vi "tipshaping.vi"(8 "error in (no error)":errorcluster, 11 "Input":string="-286.640625n,21.171875n,-1.8n,20m,200m") -> (0 "error out":errorcluster, 3 "Output":string="-7.271E-9")   [LabVIEW 2019]
panel:
  out "size(s)":i32=5
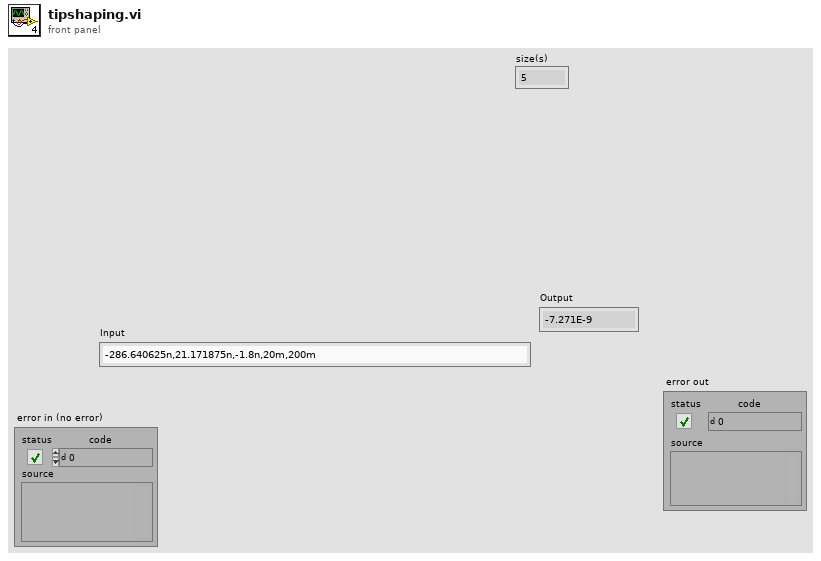
[diagram p1: front panel]
types:
  T1 = cluster{"TipLift":dbl, "Bias Settling Time":dbl, "Lift Height":dbl, "Lift Time 2":dbl, "Lifting Bias":dbl, "Lift Time 1":dbl}
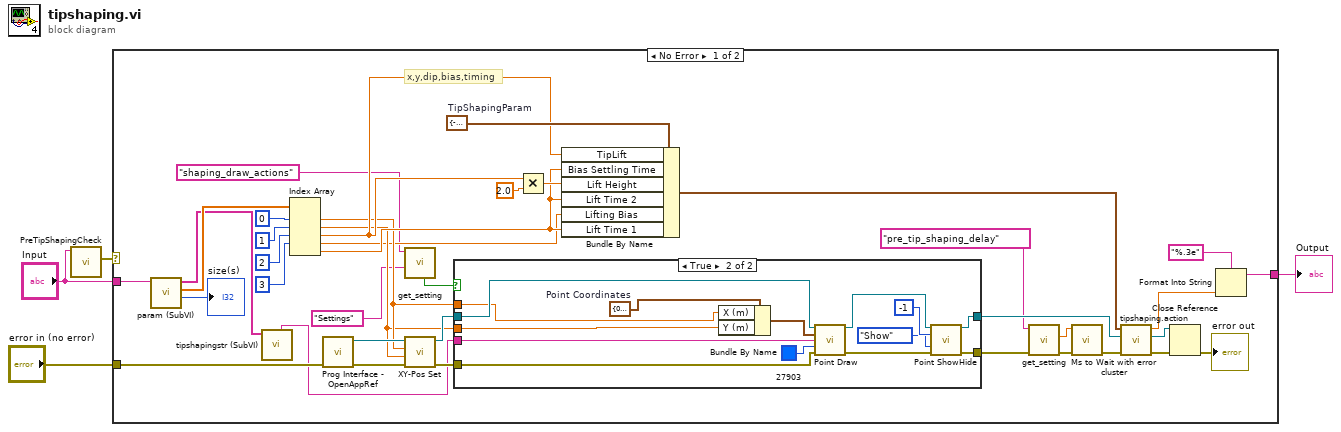
[diagram p0: block diagram]
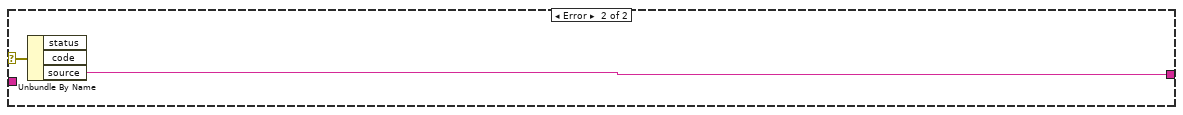
[diagram p3: hidden frame]
diagram:
  n1 = call "PreTipShapingCheck.vi"("Input"="Input") -> ("Error"=w1:errorcluster)  [unwired: 8 in, 2 out]
  n2 = case shown="No Error" w1 {
    selector: w1 -> [_ w60]
    tunnel: [w40 w59] -> w4
    tunnel: "error in (no error)" -> [w33 _]
    tunnel: "Input" -> [w18 _]
    frame No Error {
      w37 = T1 {"TipLift"=-2e-10, "Bias Settling Time"=0.09999999999999999, "Lift Height"=5e-09, "Lift Time 2"=0.2, "Lifting Bias"=2.0, "Lift Time 1"=0.2}  # TipShapingParam
      # "x,y,dip,bias,timing"
      n3 = call "param (SubVI).vi"("Input"=w18) -> ("num"=→"size(s)":i32, "parm"=w41:dbl[], "Array"=w19:string[])  [unwired: 8 in]
      n4 = call "tipshapingstr (SubVI).vi"("Array"=w19) -> ("String"=w20:string)  [unwired: 10 in]
      n5 = Index Array(array=w41, index #1=0 ("index"), index #2=1 ("index"), index #3=2 ("index"), index #4=3 ("index")) -> (element #1=w26:dbl, element #2=w25:dbl, element #3=w32:dbl, element #4=w13:dbl, element #5=w29:dbl)  [unwired: 1 in]
      n6 = call <userlib>:"Prog Interface - OpenAppRef.vi"("Error in (no error)"=w33) -> ("Error out"=w34:errorcluster, "Application reference"=w35:refnum<vi>)  [unwired: 5 in]
      n7 = call "get_setting.vi"("section"="Settings", "key"="shaping_draw_actions") -> ("Boolean"=w5:bool)  [unwired: 5 in, 4 out]
      n8 = call <userlib>:"XY-Pos Set.vi"("error in (no error)"=w34, "Y (m)"=w25, "X (m)"=w26, "Application ref in"=w35) -> ("error out"=w27:errorcluster, "Application ref out"=w28:refnum<vi>)  [unwired: 4 in]
      n9 = case shown="True" w5 {
        tunnel: w28 -> [w44 w58]
        tunnel: [w44 w55] -> w17
        tunnel: w27 -> [w43 w57]
        tunnel: [w43 w54] -> w11
        tunnel: w26 -> [_ w47]
        tunnel: w25 -> [_ w46]
        tunnel: w20 -> [_ w45]
        frame False {
        }
        frame True {
          w49 = cluster{"X (m)":sgl, "Y (m)":sgl} {"X (m)"=0.0, "Y (m)"=0.0}  # Point Coordinates
          n10 = Bundle By Name(cluster=w49, "X (m)"=w47, "Y (m)"=w46) -> (w48:cluster{"X (m)":sgl, "Y (m)":sgl})
          n11 = call <userlib>:"Point Draw.vi"("Application ref in"=w58, "Point Coordinates"=w48, "Text"=w45, "Color"=u32 27903, "error in (no error)"=w57) -> ("Application ref out"=w56:refnum<vi>, "error out"=w53:errorcluster)  [unwired: 9 in]
          n12 = call <userlib>:"Point ShowHide.vi"("Application ref in"=w56, "Point index (-1=All points)"=-1, "Show/Hide"=enum16{"Show", "Hide"}."Show", "error in (no error)"=w53) -> ("Application ref out"=w55:refnum<vi>, "error out"=w54:errorcluster)  [unwired: 10 in]
        }
      }
      n13 = Multiply(x=w32, y=2.0) -> (x*y=w31:dbl)
      n14 = Bundle By Name(cluster=w37, "TipLift"=w32, "Bias Settling Time"=w29, "Lift Height"=w31, "Lift Time 2"=w29, "Lifting Bias"=w13, "Lift Time 1"=w29) -> (w36:T1)
      n15 = call "get_setting.vi"("error in (no error)"=w11, "key"="pre_tip_shaping_delay") -> ("error out"=w10:errorcluster, "output 1"=w9:dbl)  [unwired: 5 in, 3 out]
      n16 = call <userlib>:"Ms to Wait with error cluster.vi"("error in (no error)"=w10, "milliseconds to wait"=w9) -> ("error out"=w12:errorcluster)  [unwired: 4 in, 1 out]
      n17 = call "tipshaping.action.vi"("Error in (no error)"=w12, "Application reference"=w17, "TipShapingParam"=w36) -> ("error out"=w15:errorcluster, "Application ref out"=w16:refnum<vi>, "dz"=w39:sgl)  [unwired: 6 in]
      n18 = Close Reference(reference=w16, error in (no error)=w15) -> (error out=→"error out":errorcluster)
      n19 = Format Into String(format string="%.3e", w39) -> (resulting string=w40:string)  [unwired: 2 in, 1 out]
    }
    frame Error {
      n20 = Unbundle By Name(w60) -> ("source"=w59:string)  [unwired: 2 out]
    }
  }
  "Output" <- w4
